vi "GetEdgesAndNodes.vi"(5 "PythonConverter_BD in":refnum<class "PyConvBD.lvclass">, 9 "Diagram in":refnum<class "Diagram.lvclass">) -> (3 "Diagram out":refnum<class "Diagram.lvclass">, 4 "PythonConverter_BD out":refnum<class "PyConvBD.lvclass">)   [LabVIEW 2014, in "Raspberry Pi Compatible Compiler for LabVIEW.lvlib" / "Diagram.lvclass"]
uses:
  Diagram.lvclass
  Python/PythonConverter_BD/PyConvBD.lvclass
  VI_AST/VI_AST.lvclass
  Diagram.lvclass/Diagram.ctl
  Wire/Wire.lvclass/Wire.ctl
  Python/PythonConverter_BD/PyConvBD.lvclass/PyConvBD.ctl
  FlatSequence/FlatSequence.lvclass/FlatSequence.ctl
  FlatSequence/FlatSequence.lvclass
  FlatSequenceFrame/FlatSequenceFrame.lvclass
  Wire/Wire.lvclass
  VI Interpreter/VI Interpreter.lvclass
  Tunnel/Tunnel.lvclass
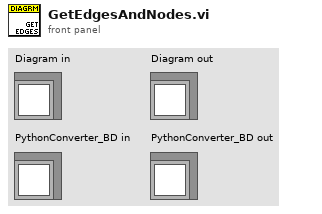
[diagram p1: front panel]
types:
  T1 = typedef "Raspberry Pi Compatible Compiler for LabVIEW.lvlib/ConnectionsTD.ctl" = cluster{"source":refnum<class "Terminal.lvclass">, "sink":refnum<class "Terminal.lvclass">}
  T2 = typedef "Raspberry Pi Compatible Compiler for LabVIEW.lvlib/VI Interpreter.lvclass/connectionType_TD.ctl" = enum16{"outer tunnel", "inner tunnel", "FSS outer tunnel", "FSS inner tunnel", "node"}
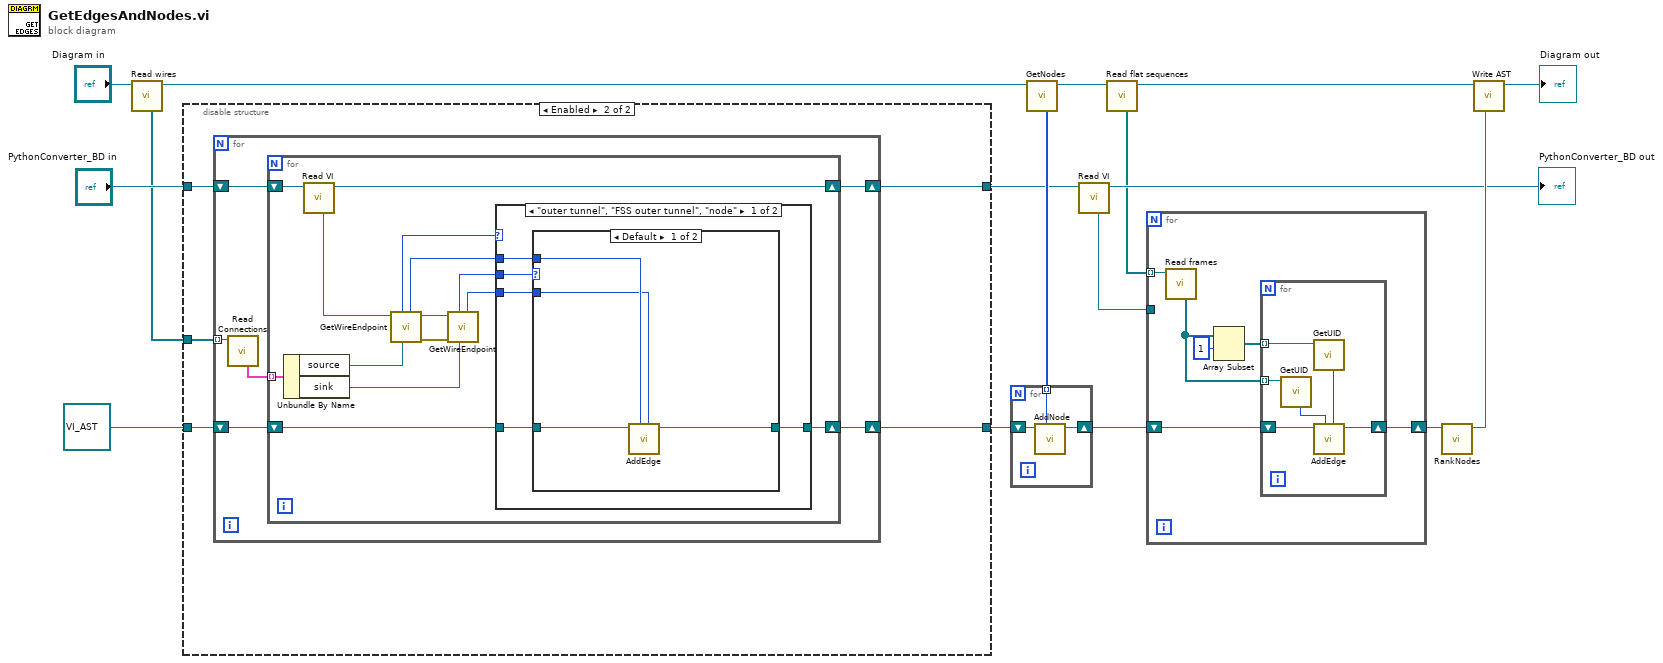
[diagram p0: block diagram]
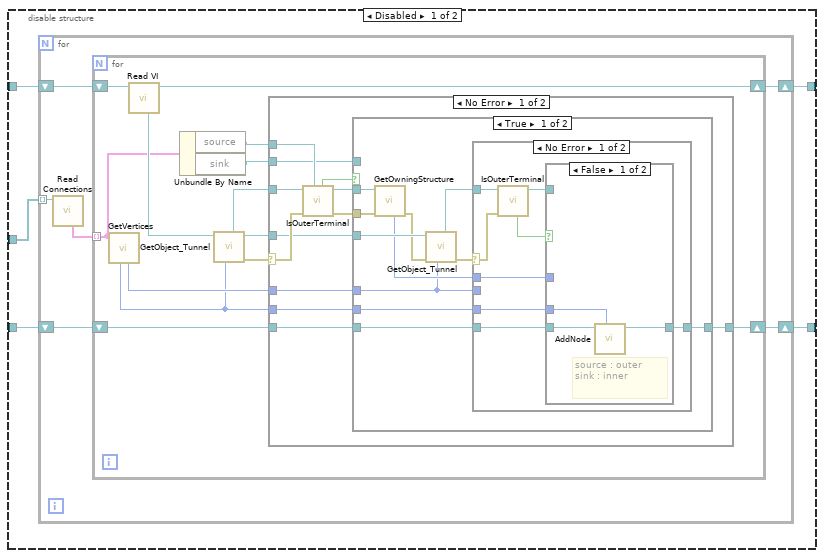
[diagram p2: hidden frame]
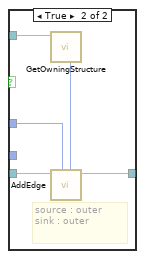
[diagram p3: hidden frame]
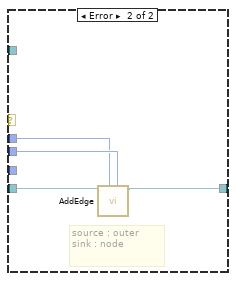
[diagram p4: hidden frame]
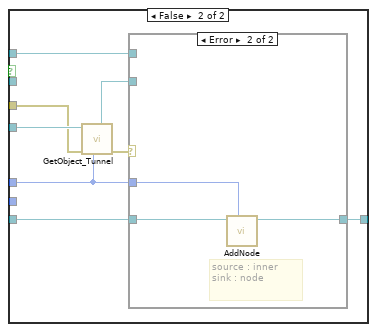
[diagram p5: hidden frame]
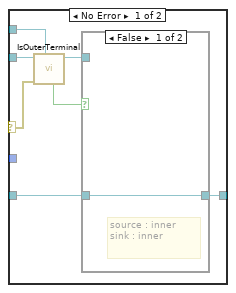
[diagram p6: hidden frame]
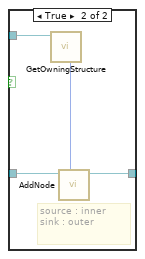
[diagram p7: hidden frame]
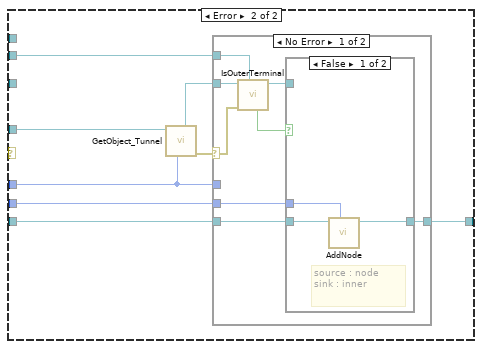
[diagram p8: hidden frame]
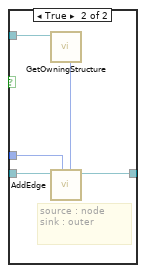
[diagram p9: hidden frame]
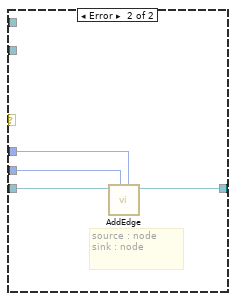
[diagram p10: hidden frame]
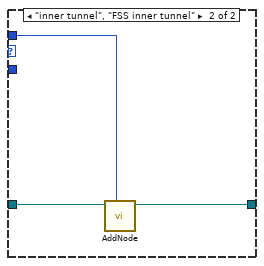
[diagram p11: hidden frame]
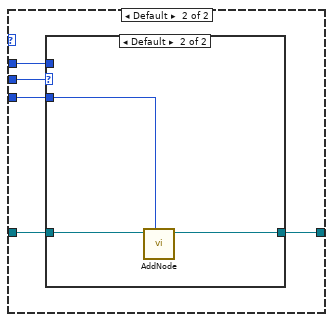
[diagram p12: hidden frame]
diagram:
  n1 = call "Read wires.vi"("Diagram in"="Diagram in") -> ("Diagram out"=w13:refnum<class "Diagram.lvclass">, "wires"=w14:refnum<class "Wire.lvclass">[])  [unwired: 7 in]
  n2 = disable-structure shown="Enabled" {
    disable-tunnel: [w22 w140] -> w6
    disable-tunnel: "PythonConverter_BD in" -> [w21 w139]
    disable-tunnel: refnum<class "VI_AST.lvclass"> refnum ("VI_AST.lvclass") -> [w20 w138]
    disable-tunnel: w14 -> [w19 w137]
    disable-tunnel: [w18 w136] -> w12
    frame Disabled {
      n3 = for {
        tunnel: w19 -> [w28] mode=indexing
        shift-right: [w25] -> w18
        shift-left: w20 -> [w26]
        shift-right: [w23] -> w22
        shift-left: w21 -> [w24]
        n4 = call "Read Connections.vi"("Wire in"=w28) -> ("Connections"=w27:T1[])  [unwired: 7 in, 1 out]
        n5 = for {
          tunnel: w27 -> [w31] mode=indexing
          shift-right: [w34] -> w25
          shift-left: w26 -> [w35]
          shift-right: [w40] -> w23
          shift-left: w24 -> [w41]
          n6 = call "GetVertices.vi"("connection"=w31) -> ("sink UID"=w37:i32, "source UID"=w32:i32)  [unwired: 5 in, 2 out]
          n7 = call "Read VI.vi"("PythonConverter_BD in"=w41) -> ("PythonConverter_BD out"=w40:refnum<class "PyConvBD.lvclass">, "VI Interpreter"=w39:refnum<class "VI Interpreter.lvclass">)  [unwired: 7 in]
          n8 = Unbundle By Name(w31) -> ("source"=w30:refnum<class "Terminal.lvclass">, "sink"=w29:refnum<class "Terminal.lvclass">)
          n9 = call "GetObject_Tunnel.vi"("UID"=w32, "VI Interpreter in"=w39) -> ("error out"=w38:errorcluster, "VI Interpreter out"=w36:refnum<class "VI Interpreter.lvclass">, "Tunnel"=w33:refnum<class "Tunnel.lvclass">)  [unwired: 4 in, 1 out]
          n10 = case shown="No Error" w38 {
            selector: w38 -> [w52 _]
            tunnel: w37 -> [w48 w115]
            tunnel: w32 -> [w46 w109]
            tunnel: w36 -> [w47 w114]
            tunnel: w35 -> [w45 w113]
            tunnel: [w44 w112] -> w34
            tunnel: w33 -> [w53 _]
            tunnel: w30 -> [w43 _]
            tunnel: w29 -> [w42 w108]
            frame No Error {
              n11 = call "IsOuterTerminal.vi"("terminal"=w43, "error in"=w52, "Tunnel in"=w53) -> ("error out"=w49:errorcluster, "Tunnel out"=w50:refnum<class "Tunnel.lvclass">, "Outer"=w51:bool)  [unwired: 4 in]
              n12 = case shown="True" w51 {
                tunnel: w50 -> [w64 _]
                tunnel: w49 -> [w63 w87]
                tunnel: w48 -> [w55 w86]
                tunnel: w47 -> [w62 w92]
                tunnel: w46 -> [w54 _]
                tunnel: w45 -> [w58 w89]
                tunnel: [w57 w88] -> w44
                tunnel: w42 -> [_ w85]
                frame True {
                  n13 = call "GetOwningStructure.vi"("error in"=w63, "Tunnel in"=w64) -> ("error out"=w61:errorcluster, "UID"=w56:i32)  [unwired: 5 in, 1 out]
                  n14 = call "GetObject_Tunnel.vi"("UID"=w55, "error in"=w61, "VI Interpreter in"=w62) -> ("error out"=w60:errorcluster, "Tunnel"=w59:refnum<class "Tunnel.lvclass">)  [unwired: 3 in, 2 out]
                  n15 = case shown="No Error" w60 {
                    selector: w60 -> [w71 _]
                    tunnel: w59 -> [w72 _]
                    tunnel: w58 -> [w68 w84]
                    tunnel: [w67 w83] -> w57
                    tunnel: w55 -> [_ w82]
                    tunnel: w56 -> [w66 w81]
                    tunnel: w54 -> [w65 _]
                    frame No Error {
                      n16 = call "IsOuterTerminal.vi"("error in"=w71, "Tunnel in"=w72) -> ("Tunnel out"=w69:refnum<class "Tunnel.lvclass">, "Outer"=w70:bool)  [unwired: 5 in, 1 out]
                      n17 = case shown="False" w70 {
                        tunnel: w69 -> [_ w80]
                        tunnel: w68 -> [w75 w79]
                        tunnel: [w74 w78] -> w67
                        tunnel: w66 -> [_ w76]
                        tunnel: w65 -> [w73 _]
                        frame False {
                          # "source : outer\nsink : inner"
                          n18 = call "AddNode.vi"("UID"=w73, "VI_AST in"=w75) -> ("VI_AST out"=w74:refnum<class "VI_AST.lvclass">)  [unwired: 6 in, 1 out]
                        }
                        frame True {
                          # "source : outer\nsink : outer"
                          n19 = call "GetOwningStructure.vi"("Tunnel in"=w80) -> ("UID"=w77:i32)  [unwired: 6 in, 2 out]
                          n20 = call "AddEdge.vi"("sink"=w77, "source"=w76, "VI_AST in"=w79) -> ("VI_AST out"=w78:refnum<class "VI_AST.lvclass">)  [unwired: 6 in]
                        }
                      }
                    }
                    frame Error {
                      # "source : outer\nsink : node"
                      n21 = call "AddEdge.vi"("sink"=w82, "source"=w81, "VI_AST in"=w84) -> ("VI_AST out"=w83:refnum<class "VI_AST.lvclass">)  [unwired: 6 in]
                    }
                  }
                }
                frame False {
                  n22 = call "GetObject_Tunnel.vi"("UID"=w86, "error in"=w87, "VI Interpreter in"=w92) -> ("error out"=w91:errorcluster, "Tunnel"=w90:refnum<class "Tunnel.lvclass">)  [unwired: 3 in, 2 out]
                  n23 = case shown="Error" w91 {
                    selector: w91 -> [w98 _]
                    tunnel: w90 -> [w99 _]
                    tunnel: w89 -> [w95 w107]
                    tunnel: [w94 w105] -> w88
                    tunnel: w86 -> [_ w106]
                    tunnel: w85 -> [w93 _]
                    frame No Error {
                      n24 = call "IsOuterTerminal.vi"("terminal"=w93, "error in"=w98, "Tunnel in"=w99) -> ("Tunnel out"=w96:refnum<class "Tunnel.lvclass">, "Outer"=w97:bool)  [unwired: 4 in, 1 out]
                      n25 = case shown="False" w97 {
                        tunnel: w96 -> [_ w104]
                        tunnel: w95 -> [w100 w103]
                        tunnel: [w100 w102] -> w94
                        frame False {
                          # "source : inner\nsink : inner"
                        }
                        frame True {
                          # "source : inner\nsink : outer"
                          n26 = call "GetOwningStructure.vi"("Tunnel in"=w104) -> ("UID"=w101:i32)  [unwired: 6 in, 2 out]
                          n27 = call "AddNode.vi"("UID"=w101, "VI_AST in"=w103) -> ("VI_AST out"=w102:refnum<class "VI_AST.lvclass">)  [unwired: 6 in, 1 out]
                        }
                      }
                    }
                    frame Error {
                      # "source : inner\nsink : node"
                      n28 = call "AddNode.vi"("UID"=w106, "VI_AST in"=w107) -> ("VI_AST out"=w105:refnum<class "VI_AST.lvclass">)  [unwired: 6 in, 1 out]
                    }
                  }
                }
              }
            }
            frame Error {
              n29 = call "GetObject_Tunnel.vi"("UID"=w115, "VI Interpreter in"=w114) -> ("error out"=w111:errorcluster, "Tunnel"=w110:refnum<class "Tunnel.lvclass">)  [unwired: 4 in, 2 out]
              n30 = case shown="No Error" w111 {
                selector: w111 -> [w122 _]
                tunnel: w110 -> [w123 _]
                tunnel: w113 -> [w119 w135]
                tunnel: [w118 w134] -> w112
                tunnel: w115 -> [_ w133]
                tunnel: w109 -> [w117 w132]
                tunnel: w108 -> [w116 _]
                frame No Error {
                  n31 = call "IsOuterTerminal.vi"("terminal"=w116, "error in"=w122, "Tunnel in"=w123) -> ("Tunnel out"=w120:refnum<class "Tunnel.lvclass">, "Outer"=w121:bool)  [unwired: 4 in, 1 out]
                  n32 = case shown="False" w121 {
                    tunnel: w120 -> [_ w131]
                    tunnel: w119 -> [w126 w130]
                    tunnel: [w124 w128] -> w118
                    tunnel: w117 -> [w125 w127]
                    frame False {
                      # "source : node\nsink : inner"
                      n33 = call "AddNode.vi"("UID"=w125, "VI_AST in"=w126) -> ("VI_AST out"=w124:refnum<class "VI_AST.lvclass">)  [unwired: 6 in, 1 out]
                    }
                    frame True {
                      # "source : node\nsink : outer"
                      n34 = call "GetOwningStructure.vi"("Tunnel in"=w131) -> ("UID"=w129:i32)  [unwired: 6 in, 2 out]
                      n35 = call "AddEdge.vi"("sink"=w129, "source"=w127, "VI_AST in"=w130) -> ("VI_AST out"=w128:refnum<class "VI_AST.lvclass">)  [unwired: 6 in]
                    }
                  }
                }
                frame Error {
                  # "source : node\nsink : node"
                  n36 = call "AddEdge.vi"("sink"=w133, "source"=w132, "VI_AST in"=w135) -> ("VI_AST out"=w134:refnum<class "VI_AST.lvclass">)  [unwired: 6 in]
                }
              }
            }
          }
        }
      }
    }
    frame Enabled {
      n37 = for {
        tunnel: w137 -> [w146] mode=indexing
        shift-right: [w143] -> w136
        shift-left: w138 -> [w144]
        shift-right: [w141] -> w140
        shift-left: w139 -> [w142]
        n38 = call "Read Connections.vi"("Wire in"=w146) -> ("Connections"=w145:T1[])  [unwired: 7 in, 1 out]
        n39 = for {
          tunnel: w145 -> [w158] mode=indexing
          shift-right: [w147] -> w143
          shift-left: w144 -> [w148]
          shift-right: [w159] -> w141
          shift-left: w142 -> [w160]
          n40 = Unbundle By Name(w158) -> ("source"=w156:refnum<class "Terminal.lvclass">, "sink"=w153:refnum<class "Terminal.lvclass">)
          n41 = call "Read VI.vi"("PythonConverter_BD in"=w160) -> ("PythonConverter_BD out"=w159:refnum<class "PyConvBD.lvclass">, "VI Interpreter"=w157:refnum<class "VI Interpreter.lvclass">)  [unwired: 7 in]
          n42 = call "GetWireEndpoint.vi"("terminal"=w156, "VI Interpreter in"=w157) -> ("error out"=w155:errorcluster, "VI Interpreter out"=w154:refnum<class "VI Interpreter.lvclass">, "connection UID"=w151:i32, "connection type"=w152:T2)  [unwired: 6 in]
          n43 = call "GetWireEndpoint.vi"("terminal"=w153, "error in"=w155, "VI Interpreter in"=w154) -> ("connection UID"=w149:i32, "connection type"=w150:T2)  [unwired: 5 in, 2 out]
          n44 = case shown="\"outer tunnel\", \"FSS outer tunnel\", \"node\"" w152 {
            tunnel: w151 -> [w165 w177]
            tunnel: w150 -> [w164 w176]
            tunnel: w149 -> [w163 w175]
            tunnel: w148 -> [w162 w174]
            tunnel: [w161 w173] -> w147
            frame "outer tunnel", "FSS outer tunnel", "node" {
              n45 = case shown="Default" w164 {
                tunnel: w165 -> [w167 w170]
                tunnel: w163 -> [w166 _]
                tunnel: w162 -> [w169 w172]
                tunnel: [w168 w171] -> w161
                frame Default {
                  n46 = call "AddEdge.vi"("sink"=w166, "source"=w167, "VI_AST in"=w169) -> ("VI_AST out"=w168:refnum<class "VI_AST.lvclass">)  [unwired: 6 in]
                }
                frame "inner tunnel", "FSS inner tunnel" {
                  n47 = call "AddNode.vi"("UID"=w170, "VI_AST in"=w172) -> ("VI_AST out"=w171:refnum<class "VI_AST.lvclass">)  [unwired: 6 in, 1 out]
                }
              }
            }
            frame Default {
              n48 = case shown="Default" w176 {
                tunnel: w177 -> [_ _]
                tunnel: w175 -> [_ w179]
                tunnel: w174 -> [w178 w181]
                tunnel: [w178 w180] -> w173
                frame "inner tunnel", "FSS inner tunnel" {
                }
                frame Default {
                  n49 = call "AddNode.vi"("UID"=w179, "VI_AST in"=w181) -> ("VI_AST out"=w180:refnum<class "VI_AST.lvclass">)  [unwired: 6 in, 1 out]
                }
              }
            }
          }
        }
      }
    }
  }
  n50 = call "GetNodes.vi"("Diagram in"=w13) -> ("Diagram out"=w9:refnum<class "Diagram.lvclass">, "nodes"=w11:i32[])  [unwired: 6 in, 1 out]
  n51 = for {
    shift-right: [w183] -> w4
    shift-left: w12 -> [w184]
    tunnel: w11 -> [w182] mode=indexing
    n52 = call "AddNode.vi"("UID"=w182, "VI_AST in"=w184) -> ("VI_AST out"=w183:refnum<class "VI_AST.lvclass">)  [unwired: 6 in, 1 out]
  }
  n53 = call "Read VI.vi"("PythonConverter_BD in"=w6) -> ("PythonConverter_BD out"=→"PythonConverter_BD out":refnum<class "PyConvBD.lvclass">, "VI Interpreter"=w3:refnum<class "VI Interpreter.lvclass">)  [unwired: 7 in]
  n54 = call "Read flat sequences.vi"("Diagram in"=w9) -> ("Diagram out"=w7:refnum<class "Diagram.lvclass">, "flat sequences"=w2:refnum<class "FlatSequence.lvclass">[])  [unwired: 7 in]
  n55 = for {
    shift-right: [w187] -> w1
    shift-left: w4 -> [w188]
    tunnel: w3 -> [_]
    tunnel: w2 -> [w190] mode=indexing
    n56 = call "Read frames.vi"("FlatSequence in"=w190) -> ("frames"=w185:refnum<class "FlatSequenceFrame.lvclass">[])  [unwired: 7 in, 1 out]
    n57 = Array Subset(array=w185, index=1) -> (w186:refnum<class "FlatSequenceFrame.lvclass">[])  [unwired: 1 in]
    n58 = for {
      shift-right: [w195] -> w187
      shift-left: w188 -> [w196]
      tunnel: w186 -> [w191] mode=indexing
      tunnel: w185 -> [w194] mode=indexing
      n59 = call-dynamic "GetUID.vi"("FlatSequenceFrame in"=w194) -> ("UID"=w193:i32)  [unwired: 6 in, 2 out]
      n60 = call-dynamic "GetUID.vi"("FlatSequenceFrame in"=w191) -> ("UID"=w192:i32)  [unwired: 6 in, 2 out]
      n61 = call "AddEdge.vi"("sink"=w192, "source"=w193, "VI_AST in"=w196) -> ("VI_AST out"=w195:refnum<class "VI_AST.lvclass">)  [unwired: 6 in]
    }
  }
  n62 = call "RankNodes.vi"("VI_AST in"=w1) -> ("VI_AST out"=w8:refnum<class "VI_AST.lvclass">)  [unwired: 8 in]
  n63 = call "Write AST.vi"("AST"=w8, "Diagram in"=w7) -> ("Diagram out"=→"Diagram out":refnum<class "Diagram.lvclass">)  [unwired: 7 in]
